vi "Sync.vi"(8 "error in (no error)":errorcluster, 10 "file ref":refnum<file>, 11 "size trigger in":refnum<class "RolloverTrigger.Size.lvclass">) -> (0 "error out":errorcluster, 3 "size trigger out":refnum<class "RolloverTrigger.Size.lvclass">)   [LabVIEW 2018, in "GLog.lvlib" / "RolloverTrigger.Size.lvclass"]
doc: "Resets the current file size counter to the size of the new file."
uses:
  RolloverTrigger.Size.lvclass
  RolloverTrigger.Size.lvclass/RolloverTrigger.Size.ctl
panel:
  # "Connector Pane"
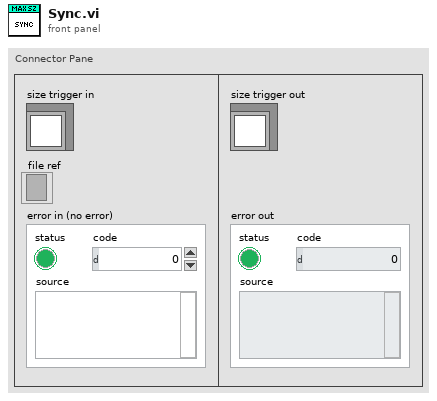
[diagram p1: front panel]
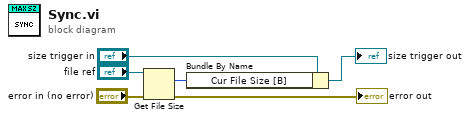
[diagram p0: block diagram]
diagram:
  n1 = Get File Size(file="file ref", error in="error in (no error)") -> (size (in bytes)=w5:i64, 0:→"error out":errorcluster)  [unwired: 1 out]
  n2 = Bundle By Name(cluster="size trigger in", "Cur File Size [B]"=w5) -> (→"size trigger out":refnum<class "RolloverTrigger.Size.lvclass">)
